vi "stop.vi"(8 "error in (no error)":errorcluster, 11 "QuadraturePositionDecoder in":refnum<class "QuadraturePositionDecoder.lvclass">) -> (0 "error out":errorcluster, 3 "QuadraturePositionDecoder out":refnum<class "QuadraturePositionDecoder.lvclass">)   [LabVIEW 2014, in "QuadraturePositionDecoder.lvclass"]
uses:
  QuadraturePositionDecoder.lvclass
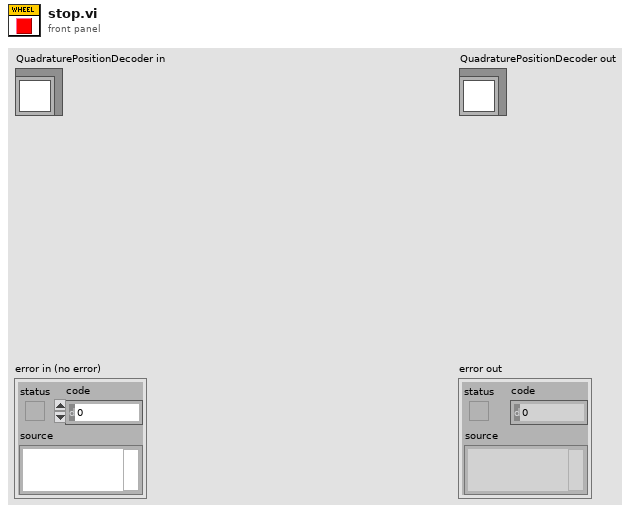
[diagram p1: front panel]
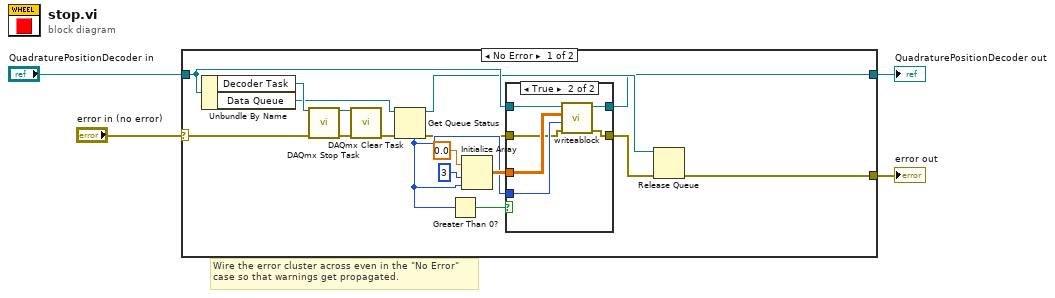
[diagram p0: block diagram]
diagram:
  # "Wire the error cluster across even in the \"No Error\"\ncase so that warnings get propagated."
  n1 = case shown="No Error" "error in (no error)" {
    selector: "error in (no error)" -> [w20 w31]
    tunnel: [w5 w31] -> w3
    tunnel: [w6 w30] -> w1
    tunnel: "QuadraturePositionDecoder in" -> [w15 w30]
    frame No Error {
      n2 = Unbundle By Name(w15) -> ("Decoder Task"=w21:refnum<k21>, "Data Queue"=w17:refnum<queue>)
      n3 = call <vilib>:"DAQmx Stop Task.vi"("task/channels in"=w21, "error in"=w20) -> ("task out"=w19:refnum<k21>, "error out"=w18:errorcluster)  [unwired: 12 in]
      n4 = call <vilib>:"DAQmx Clear Task.vi"("task in"=w19, "error in"=w18) -> ("error out"=w10:errorcluster)  [unwired: 13 in]
      n5 = Get Queue Status(queue=w17, error in (no error)=w10) -> (queue out=w8:refnum<queue>, error out=w9:errorcluster, # elements in queue=w11:i32)  [unwired: 1 in, 5 out]
      n6 = Greater Than 0?(x=w11) -> (x > 0?=w16:bool)
      n7 = Initialize Array(0.0 ("element"), 3 ("dimension size"), w11) -> (w12:dbl[][])
      n8 = case shown="True" w16 {
        tunnel: w15 -> [w23 w29]
        tunnel: [w23 w28] -> w6
        tunnel: w12 -> [_ w27]
        tunnel: w11 -> [_ w26]
        tunnel: w9 -> [w22 w25]
        tunnel: [w22 w24] -> w7
        frame False {
        }
        frame True {
          n9 = call-dynamic "writeablock.vi"("error in (no error)"=w25, "BlockSize"=w26, "Array"=w27, "QuadraturePositionDecoder in"=w29) -> ("error out"=w24:errorcluster, "QuadraturePositionDecoder out"=w28:refnum<class "QuadraturePositionDecoder.lvclass">)  [unwired: 6 in]
        }
      }
      n10 = Release Queue(queue=w8, error in (no error)=w7) -> (error out=w5:errorcluster)  [unwired: 1 in, 2 out]
    }
    frame Error {
    }
  }
  "error out" <- w3
  "QuadraturePositionDecoder out" <- w1
